vi "Read Gold Board File.vi"(11 "Application in":refnum<class "Application.lvclass">) -> (3 "Application out":refnum<class "Application.lvclass">)   [LabVIEW 2015, in "Application.lvlib" / "Application.lvclass"]
uses:
  Application.lvclass
  Application.lvclass/Application.ctl
  Properties/App Properties.lvclass/App Properties.ctl
  Properties/App Properties.lvclass
  Golden Board/Class/Golden Board.lvclass
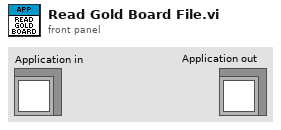
[diagram p1: front panel]
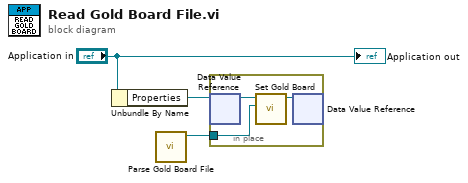
[diagram p0: block diagram]
diagram:
  n1 = Unbundle By Name("Application in") -> ("Properties"=w3:refnum<data-value>)
  n2 = call "Parse Gold Board File.vi"() -> ("Golden Board out"=w1:refnum<class "Golden Board.lvclass">)  [unwired: 10 in, 1 out]
  n3 = in-place {
    in-place-border: w1 -> [w4]
    n4 = in-place-dvr #1(w3) -> (w6:refnum<class "App Properties.lvclass">)  [unwired: 1 out]
    n5 = call "Set Gold Board.vi"("Golden Board"=w4, "App Properties in"=w6) -> ("App Properties out"=w5:refnum<class "App Properties.lvclass">)  [unwired: 8 in, 1 out]
    n6 = in-place-dvr #1(w5) -> ()  [unwired: 2 out]
  }
  "Application out" <- "Application in"
